vi "Configure Display Backlight.vi"(8 "error in (no error)":errorcluster, 10 "backlight, %":u8, 11 "VGC in":refnum<class "PL Inficon VGC.lvclass">) -> (0 "error out":errorcluster, 2 "backlight, %":u8, 3 "VGC out":refnum<class "PL Inficon VGC.lvclass">)   [LabVIEW 2015, in "PL Inficon VGC.lvclass"]
doc: "Configures display backlight."
uses:
  PL Inficon VGC.lvclass
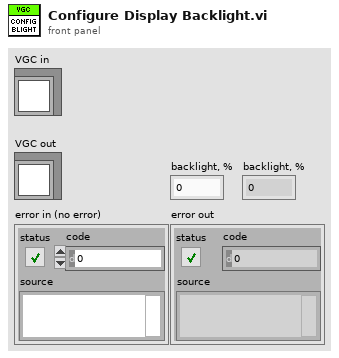
[diagram p1: front panel]
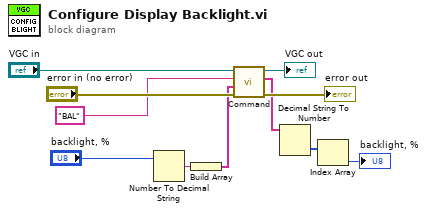
[diagram p0: block diagram]
diagram:
  n1 = Number To Decimal String(number="backlight, %") -> (decimal integer string=w7:string)  [unwired: 1 in]
  n2 = Build Array(w7) -> (w6:string[])
  n3 = call "Command.vi"("error in (no error)"="error in (no error)", "parameters"=w6, "command"="BAL" ("format string"), "VGC in"="VGC in") -> ("error out"=→"error out":errorcluster, "response data"=w4:string[], "VGC out"=→"VGC out":refnum<class "PL Inficon VGC.lvclass">)  [unwired: 5 in]
  n4 = Decimal String To Number(string=w4) -> (number=w5:i32[])  [unwired: 2 in, 1 out]
  n5 = Index Array(array=w5) -> (element=→"backlight, %":i32)  [unwired: 1 in]
